vi "TestBasicExperiment.vi"() -> ()   [LabVIEW 2017]
panel:
  in  "DelayTime":dbl=100.0
  in  "MatrixSize":dbl=100.0
  out "Processed As Control Collection":bool
  out "TestMatrix":dbl[][](graph)
  out "error out":errorcluster
  out "ExpID":string
  out "Log":string
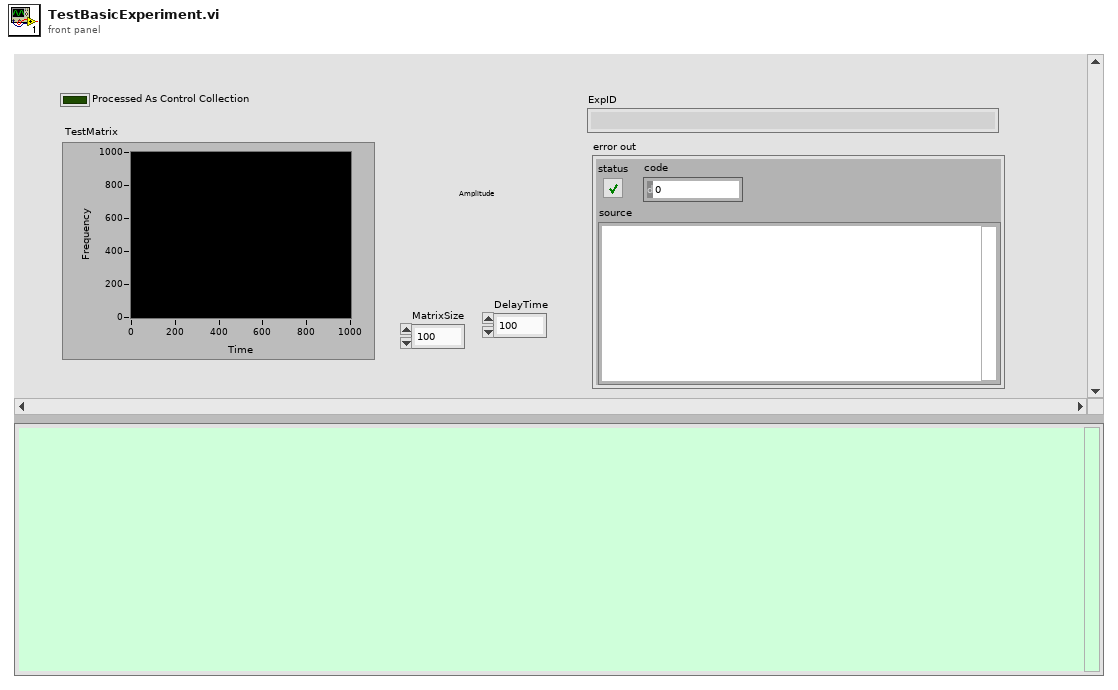
[diagram p1: front panel]
types:
  T1 = typedef "ExposeEventRegistrationDataType.ctl" = refnum<event-registration>
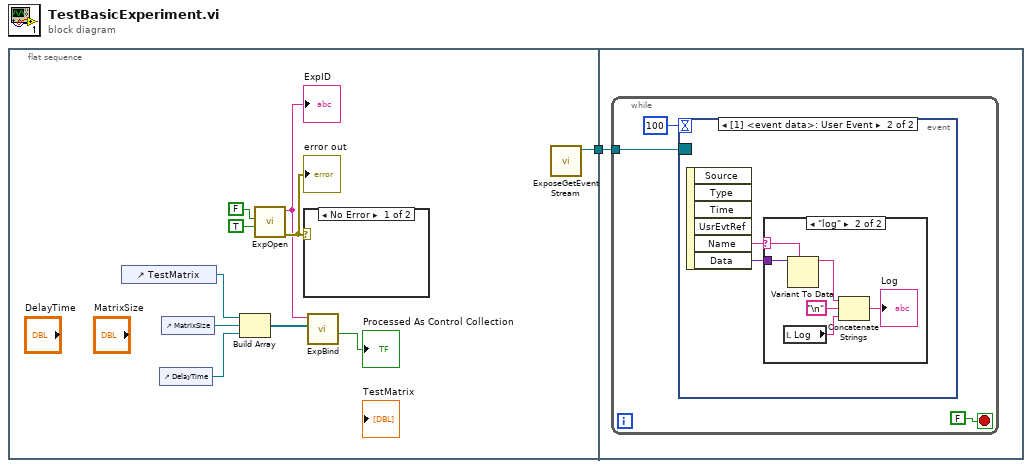
[diagram p0: block diagram]
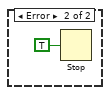
[diagram p2: hidden frame]
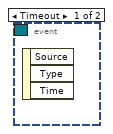
[diagram p3: hidden frame]
diagram:
  n1 = flat-sequence {
    tunnel: [w5] -> w1
    tunnel: w1 -> [w13]
    frame #0 {
      n2 = control-ref of="TestMatrix"() -> (w8:refnum<vi>)
      n3 = control-ref of="DelayTime"() -> (w2:refnum<vi>)
      n4 = control-ref of="MatrixSize"() -> (w3:refnum<vi>)
      n5 = Build Array(w8, w3, w2) -> (w7:refnum<vi>[])
      n6 = call "ExpOpen.vi"("Do Expose Logging"=TRUE, "Requires Matlab Enviroment"=FALSE) -> ("error out"=w10:errorcluster, "ExpID"=w9:string)  [unwired: 7 in, 1 out]
      "ExpID" <- w9
      "error out" <- w10
      n7 = case shown="No Error" w10 {
        frame No Error {
        }
        frame Error {
          n8 = Stop(stop? (T)=TRUE) -> ()
        }
      }
      n9 = call "ExpBind.vi"("Value"=w7, "ExpID"=w9) -> ("Processed As Control Collection"=→"Processed As Control Collection":bool)  [unwired: 9 in]
      n10 = call "ExposeGetEventStream.vi"() -> ("Event Registration Refnum out"=w5:T1)  [unwired: 8 in, 3 out]
    }
    frame #1 {
      n11 = while {
        tunnel: w13 -> [w14]
        stop <- FALSE stop-if-true
        n12 = event shown="[1] <event data>: User Event" {
          selector: w14 -> [_ _]
          dyn-events: _ -> [_ _]
          timeout: 100 -> [_ _]
          event Timeout {
            n13 = event-data() -> ()  [unwired: 1 in, 3 out]
          }
          event User Event {
            n14 = event-data() -> ("Name"=w18:string, "Data"=w17:variant)  [unwired: 1 in, 4 out]
            n15 = case shown="\"log\"" w18 {
              selector: w18 -> [_ w23]
              tunnel: w17 -> [_ w24]
              frame "False", Default {
              }
              frame "log" {
                n16 = local read "Log"() -> (w21:string)
                n17 = Variant To Data(type=w23, Variant=w24) -> (data=w22:string)  [unwired: 1 in, 1 out]
                n18 = Concatenate Strings(w22, "\n", w21) -> (→"Log":string)
              }
            }
          }
        }
      }
    }
  }
